vi "Create XML Text.vi"(0 "VIA CFG Data":T1 {"Test Configuration"."Test Ranking" items=["Low", "Normal", "High"]}) -> (4 "XML":string)   [LabVIEW 2020]
uses:
  <vilib>/addons/analyzer/Typedefs/VIACFGExport.ctl
  <vilib>/addons/analyzer/_analyzerctrls.llb/VIAnCtl TestRanking.ctl
  <vilib>/addons/analyzer/_analyzerctrls.llb/VIAnCtl Config Control Value.ctl
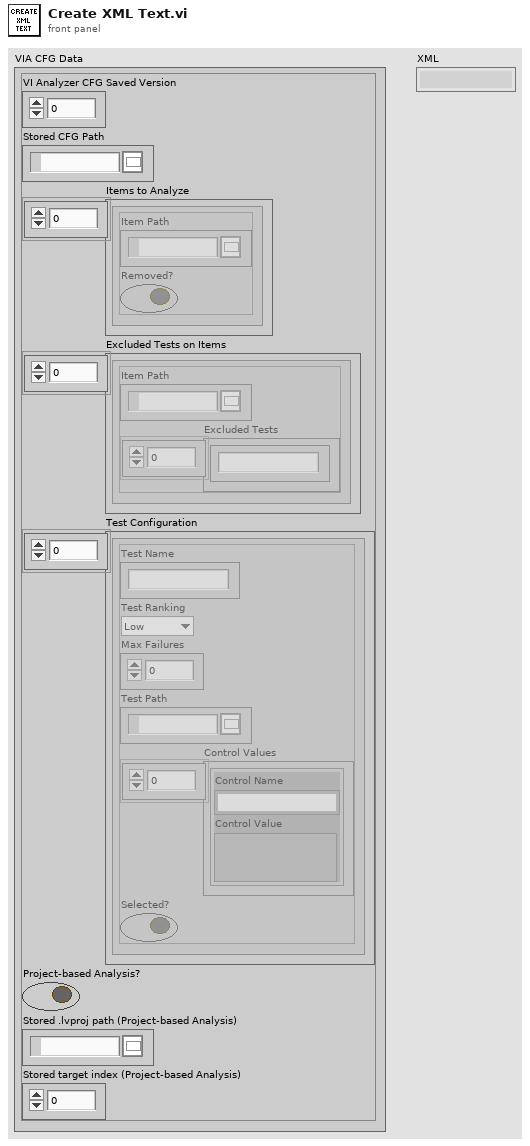
[diagram p1: front panel]
types:
  T1 = typedef "VIACFGExport.ctl" = cluster{"VI Analyzer CFG Saved Version":u16, "Stored CFG Path":path, "Items to Analyze":cluster{"Item Path":path, "Removed?":bool}[], "Excluded Tests on Items":cluster{"Item Path":path, "Excluded Tests":string[]}[], "Test Configuration":cluster{"Test Name":string, "Test Ranking":T2, "Max Failures":u32, "Test Path":path, "Control Values":T3[], "Selected?":bool}[], "Project-based Analysis?":bool, "Stored .lvproj path (Project-based Analysis)":path, "Stored target index (Project-based Analysis)":u16}
  T2 = typedef "VIAnCtl TestRanking.ctl" = u16
  T3 = typedef "VIAnCtl Config Control Value.ctl" = cluster{"Control Name":string, "Control Value":variant}
  T4 = cluster{"Item Path":path, "Excluded Tests":string[]}[]
  T5 = cluster{"Test Name":string, "Test Ranking":T2, "Max Failures":u32, "Test Path":path, "Control Values":T3[], "Selected?":bool}[]
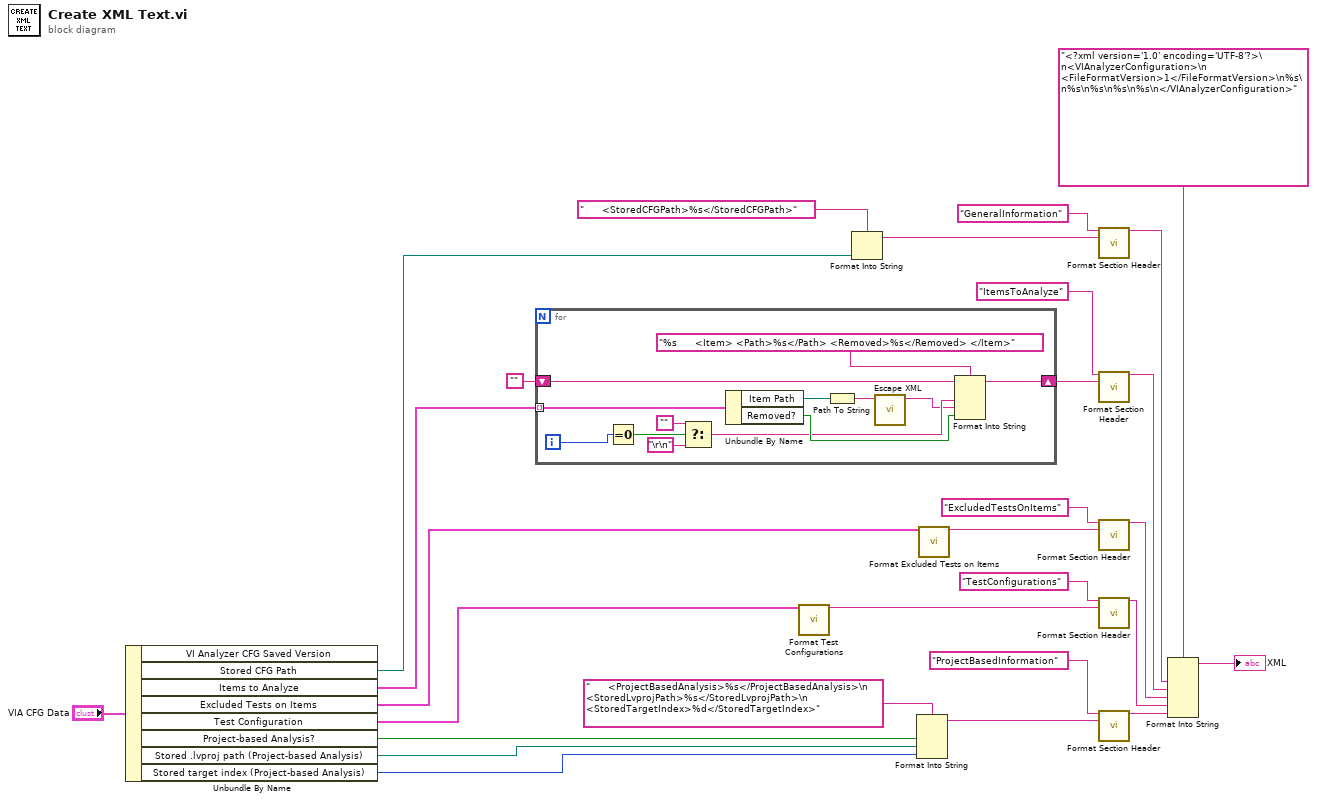
[diagram p0: block diagram]
diagram:
  n1 = Unbundle By Name("VIA CFG Data") -> ("Stored CFG Path"=w17:path, "Items to Analyze"=w2:cluster{"Item Path":path, "Removed?":bool}[], "Excluded Tests on Items"=w3:T4, "Test Configuration"=w9:T5, "Project-based Analysis?"=w25:bool, "Stored .lvproj path (Project-based Analysis)"=w26:path, "Stored target index (Project-based Analysis)"=w27:u16)  [unwired: 1 out]
  n2 = for {
    tunnel: w2 -> [w41] mode=indexing
    shift-right: [w40] -> w19
    shift-left: "" -> [w31]
    i -> [w37]
    n3 = Equal To 0?(x=w37) -> (x = 0?=w36:bool)
    n4 = Select(t="", s=w36, f="\r\n") -> (s? t:f=w32:string)
    n5 = Unbundle By Name(w41) -> ("Item Path"=w33:path, "Removed?"=w38:bool)
    n6 = Path To String(path=w33) -> (string=w29:string)
    n7 = call <vilib>:"Escape XML.vi"("XML String In"=w29) -> ("XML String Out"=w30:string)  [unwired: 9 in, 1 out]
    n8 = Format Into String(format string="%s      <Item> <Path>%s</Path> <Removed>%s</Removed> </Item>", initial string=w31, w32, w30, w38) -> (resulting string=w40:string)  [unwired: 1 in, 1 out]
  }
  n9 = call <vilib>:"Format Test Configurations.vi"("Test Configuration"=w9) -> ("formatted string"=w23:string)  [unwired: 14 in]
  n10 = Format Into String(format string="      <StoredCFGPath>%s</StoredCFGPath>", w17) -> (resulting string=w16:string)  [unwired: 2 in, 1 out]
  n11 = Format Into String(format string="      <ProjectBasedAnalysis>%s</ProjectBasedAnalysis>\n      <StoredLvprojPath>%s</StoredLvprojPath>\n      <StoredTargetIndex>%d</StoredTargetIndex>", w25, w26, w27) -> (resulting string=w28:string)  [unwired: 2 in, 1 out]
  n12 = call <vilib>:"Format Excluded Tests on Items.vi"("excluded tests on items"=w3) -> ("formatted string"=w22:string)  [unwired: 14 in]
  n13 = call <vilib>:"Format Section Header.vi"("header"="GeneralInformation", "body"=w16) -> ("formatted section header"=w7:string)  [unwired: 13 in]
  n14 = call <vilib>:"Format Section Header.vi"("header"="ItemsToAnalyze", "body"=w19) -> ("formatted section header"=w18:string)  [unwired: 13 in]
  n15 = call <vilib>:"Format Section Header.vi"("header"="ExcludedTestsOnItems", "body"=w22) -> ("formatted section header"=w21:string)  [unwired: 13 in]
  n16 = call <vilib>:"Format Section Header.vi"("header"="TestConfigurations", "body"=w23) -> ("formatted section header"=w11:string)  [unwired: 13 in]
  n17 = call <vilib>:"Format Section Header.vi"("header"="ProjectBasedInformation", "body"=w28) -> ("formatted section header"=w13:string)  [unwired: 13 in]
  n18 = Format Into String(format string="<?xml version='1.0' encoding='UTF-8'?>\n<VIAnalyzerConfiguration>\n   <FileFormatVersion>1</FileFormatVersion>\n%s\n%s\n%s\n%s\n%s\n</VIAnalyzerConfiguration>", w7, w18, w21, w11, w13) -> (resulting string=→"XML":string)  [unwired: 2 in, 1 out]
